vi "Notifer-Ext.vi"() -> ()   [LabVIEW 2021]
doc: "Use this template to build a master/slave design pattern. The master loop always executes. It notifies one or more slave loops to execute their code. The slave loop(s) continue executing until they complete, then wait for another notification. Contrast this with the Producer/Consumer pattern in which the consumer loops execute only when they have data in their queue."
panel:
  in  "Pause":bool
  in  "Start":bool
  in  "Exit":bool
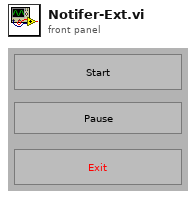
[diagram p1: front panel]
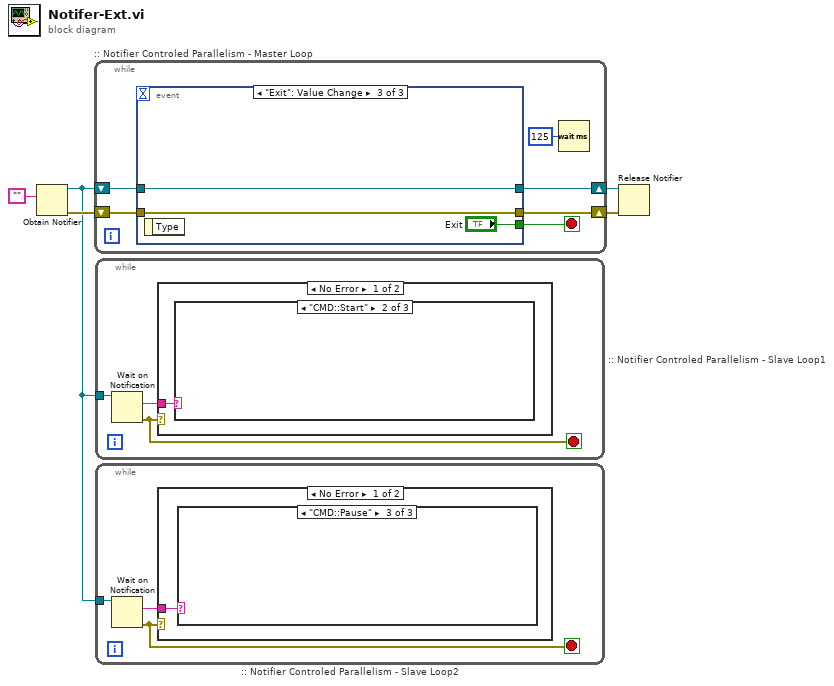
[diagram p0: block diagram]
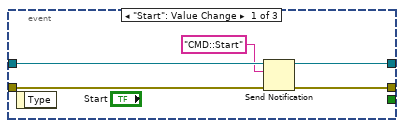
[diagram p8: hidden frame]
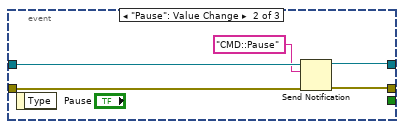
[diagram p9: hidden frame]
diagram:
  n1 = Obtain Notifier(notification data type="" ("data (can be any type)")) -> (notifier out=w1:refnum<notifier>, error out=w5:errorcluster)  [unwired: 2 in, 2 out]
  n2 = while ":: Notifier Controled Parallelism - Master Loop" {
    shift-right: [w10] -> w4
    shift-left: w5 -> [w9]
    shift-right: [w8] -> w3
    shift-left: w1 -> [w11]
    stop <- w6 stop-if-true
    n3 = event shown="[2] \"Exit\": Value Change" {
      selector: _ -> [_ _ _]
      dyn-events: _ -> [_ _ _]
      timeout: _ -> [_ _ _]
      tunnel: w11 -> [w16 w21 w24]
      tunnel: [w15 w17 w23] -> w10
      tunnel: w9 -> [w14 w18 w23]
      tunnel: [w13 w19 w24] -> w8
      tunnel: [_ _ "Exit"] -> w6
      event "Start": Value Change {
        n4 = event-data() -> ()  [unwired: 1 in, 1 out]
        n5 = Send Notification(notification="CMD::Start", notifier=w16, error in (no error)=w14) -> (notifier out=w13:refnum<notifier>, error out=w15:errorcluster)
      }
      event "Pause": Value Change {
        n6 = event-data() -> ()  [unwired: 1 in, 1 out]
        n7 = Send Notification(notification="CMD::Pause", notifier=w21, error in (no error)=w18) -> (notifier out=w19:refnum<notifier>, error out=w17:errorcluster)
      }
      event "Exit": Value Change {
        n8 = event-data() -> ()  [unwired: 1 in, 1 out]
      }
    }
    n9 = Wait (ms)(milliseconds to wait=u32 125) -> ()  [unwired: 1 out]
  }
  n10 = while ":: Notifier Controled Parallelism - Slave Loop1" {
    tunnel: w1 -> [w27]
    stop <- w26 stop-if-true
    n11 = Wait on Notification(notifier=w27) -> (notification=w25:string, error out=w26:errorcluster)  [unwired: 1 in, 4 out]
    n12 = case shown="No Error" w26 {
      tunnel: w25 -> [w28 _]
      frame No Error {
        n13 = case shown="\"CMD::Start\"" w28 {
          frame Default {
          }
          frame "CMD::Start" {
          }
          frame "CMD::Pause" {
          }
        }
      }
      frame Error {
      }
    }
  }
  n14 = while ":: Notifier Controled Parallelism - Slave Loop2" {
    tunnel: w1 -> [w31]
    stop <- w30 stop-if-true
    n15 = Wait on Notification(notifier=w31) -> (notification=w29:string, error out=w30:errorcluster)  [unwired: 1 in, 4 out]
    n16 = case shown="No Error" w30 {
      tunnel: w29 -> [w32 _]
      frame No Error {
        n17 = case shown="\"CMD::Pause\"" w32 {
          frame Default {
          }
          frame "CMD::Start" {
          }
          frame "CMD::Pause" {
          }
        }
      }
      frame Error {
      }
    }
  }
  n18 = Release Notifier(notifier=w3, error in (no error)=w4) -> ()  [unwired: 4 out]
